vi "Close_Data_Trans_Ref.vi"() -> (0 "Error Out":errorcluster)   [LabVIEW 2010]
uses:
  DataTranslation_global.vi
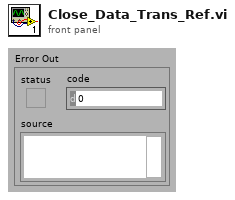
[diagram p1: front panel]
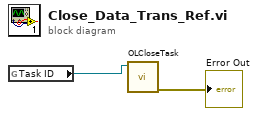
[diagram p0: block diagram]
diagram:
  n1 = global read "DataTranslation_global.vi" "Task ID"() -> (w2:refnum<k24>)
  n2 = call "OLCloseTask.vi"("Task In"=w2) -> ("Error Out"=→"Error Out":errorcluster)  [unwired: 10 in]
